vi "WPI_CameraGet Frame Rate.vi"(8 "error in (no error)":errorcluster, 11 "CameraDevRef":T2) -> (0 "error out":errorcluster, 2 "Frame Rate (fps)":T1, 3 "CameraDevRef Out":T2)   [LabVIEW 2017]
doc: "Returns the frequency, in frames per second, at which the camera you specify captures a new set of image data.\n\nThis software is licensed. Open the labview\\readme\\WPI Robotics Library Open Source License.txt file for more information."
uses:
  <vilib>/Rock Robotics/WPI/Camera/WPI_CameraDevRef.ctl
  <vilib>/Rock Robotics/WPI/Camera/WPI_CameraFrameRate.ctl
  <vilib>/Rock Robotics/WPI/Camera/WPI_CameraSettings Operations.ctl
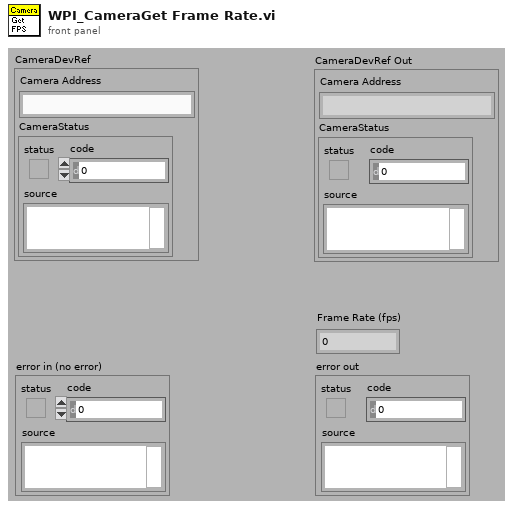
[diagram p1: front panel]
types:
  T1 = typedef "WPI_CameraFrameRate.ctl" = u32
  T2 = typedef "WPI_CameraDevRef.ctl" = cluster{"Camera Address":string, "CameraStatus":errorcluster}
  T3 = typedef "WPI_CameraSettings Operations.ctl" = enum16{"Udate FPS", "Update Compression", "Update Size", "Update White Balance", "Update Brightness", "Update Sharpness", "Update Exposure", "Update Exposure Value", "Update Color Level", "Update Exp Priority", "Update Color Enable", "Update JPG", "Update MJPG", "Read and Clear", "Read", "Init"}
  T4 = typedef "WPI_CameraSettings Control.ctl" = cluster{"FPS":i32, "Compression":i32, "Size":i32, "White Balance":i32, "Brightness":i32, "Sharpness":i32, "Exposure":i32, "Color Level":i32, "Exposure Priority":i32, "Color Enable":i32, "JPG Loop":i32, "MJPG Loop":i32, "Exposure Value":i32}
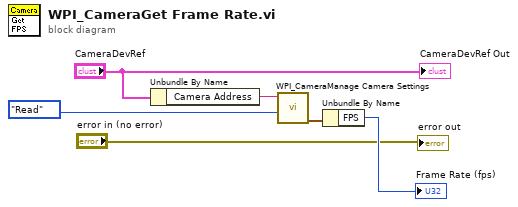
[diagram p0: block diagram]
diagram:
  n1 = Unbundle By Name("CameraDevRef") -> ("Camera Address"=w5:string)
  n2 = call <vilib>:"WPI_CameraManage Camera Settings.vi"("Operation"=WPI_CameraSettings_Operations."Read", "Camera IP"=w5) -> ("Values"=w3:T4)  [unwired: 8 in, 1 out]
  n3 = Unbundle By Name(w3) -> ("FPS"=→"Frame Rate (fps)":i32)
  "CameraDevRef Out" <- "CameraDevRef"
  "error out" <- "error in (no error)"
